vi "FitLinear2 (SubVI).vi"(0 "x values":dbl[](array[numeric]), 1 "y values":dbl[](array[numeric]), 2 "delta y values":dbl[](array[numeric]), 4 "confidence level":dbl=0.95, 5 "error in":errorcluster, 6 "Use all points":bool, 7 "Estimated centre":dbl, 8 "Fit method":T1 items=["Least Square", "Least Absolute Residual", "Bisquare"], 9 "Estimated width":dbl, 10 "Fit parameter bounds":T2={"slope min"=-inf, "slope max"=inf, "intercept min"=-inf, "intercept max"=inf}, 11 "Nsigma Low":dbl=4.0 format="%#_13g", 13 "Nsigma High":dbl=4.0 format="%#_13g") -> (14 "slope":dbl, 15 "delta slope":dbl, 16 "intercept":dbl, 17 "delta intercept":dbl, 18 "Plot with linear fit":T3(graph), 19 "error out":errorcluster)   [LabVIEW 2016]
uses:
  <vilib>/Analysis/6fits.llb/Curve Fitting Criteria.ctl
  <vilib>/Analysis/6fits.llb/Confidence Interval (Linear).vi
  <vilib>/Analysis/NI_AALPro.lvlib
panel:
  out "Best Linear Fit":dbl[](array[numeric])
  out "Selected y values":dbl[](array[numeric])
  out "Selected x values":dbl[](array[numeric])
  out "Selected delta y values":dbl[](array[numeric])
  out "residue":dbl
  # "RESULTS"
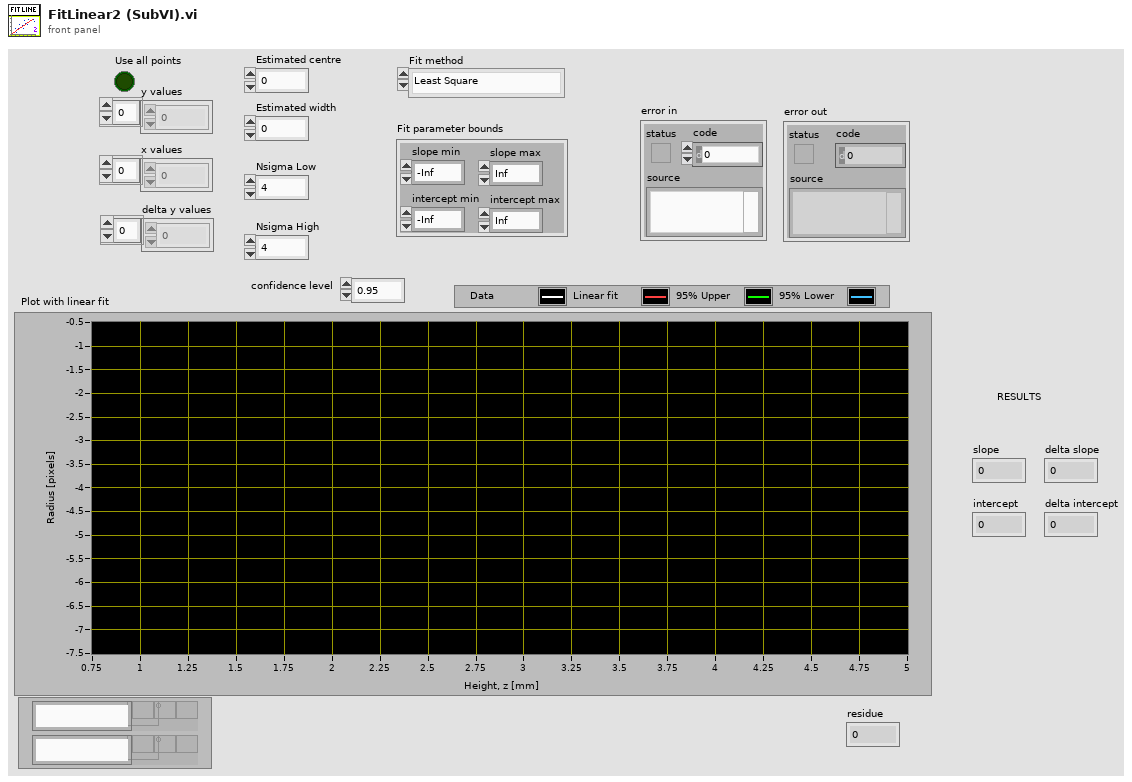
[diagram p1: front panel]
types:
  T1 = typedef "NI_AALPro.lvlib/Curve Fitting Criteria.ctl" = u16
  T2 = cluster{"slope min":dbl, "slope max":dbl, "intercept min":dbl, "intercept max":dbl}
  T3 = cluster{"Radius bins":dbl[], "Best Gaussian Fit":dbl[]}[]
  T4 = cluster{"Selected x values":dbl[], "Selected y values":dbl[]}
  T5 = cluster{"Selected x values":dbl[], "Best Linear Fit":dbl[]}
  T6 = cluster{"Selected x values":dbl[], "Upper Bound":dbl[]}
  T7 = cluster{"Selected x values":dbl[], "Lower Bound":dbl[]}
  T8 = cluster{"Selected x values":dbl[], "Lower Bound":dbl[]}[]
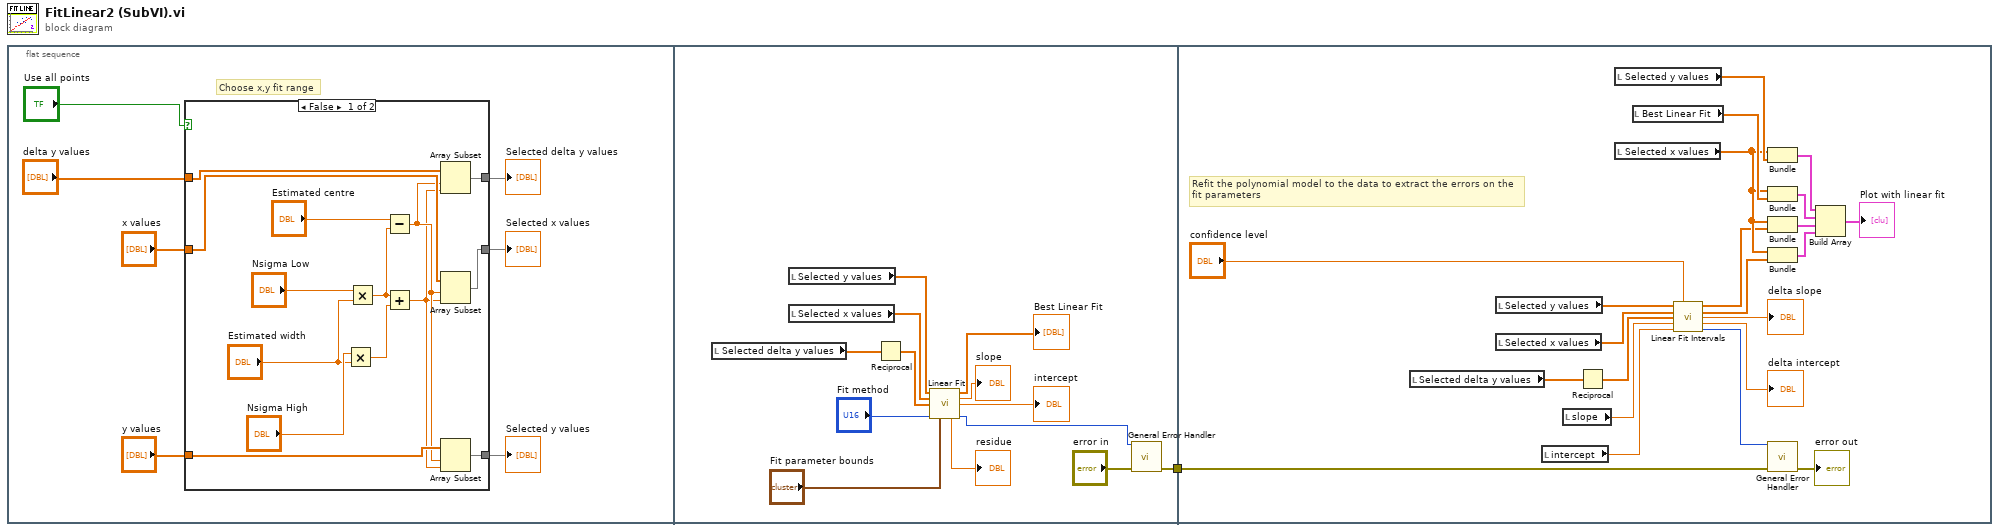
[diagram p0: block diagram]
diagram:
  n1 = flat-sequence {
    tunnel: [w38] -> w1
    tunnel: w1 -> [w51]
    frame #0 {
      # "Choose x,y fit range"
      n2 = case shown="False" "Use all points" {
        tunnel: "y values" -> [w20 w24]
        tunnel: [w19 w24] -> w4
        tunnel: "x values" -> [w18 w25]
        tunnel: [w17 w25] -> w5
        tunnel: "delta y values" -> [w12 w23]
        tunnel: [w9 w23] -> w2
        frame False {
          n3 = Multiply(x="Nsigma High", y="Estimated width") -> (x*y=w13:dbl)
          n4 = Multiply(x="Nsigma Low", y="Estimated width") -> (x*y=w14:dbl)
          n5 = Subtract(x="Estimated centre", y=w14) -> (x-y=w11:dbl)
          n6 = Add(x=w14, y=w13) -> (x+y=w10:dbl)
          n7 = Array Subset(array=w12, index=w11, length=w10) -> (w9:dbl[])
          n8 = Array Subset(array=w18, index=w11, length=w10) -> (w17:dbl[])
          n9 = Array Subset(array=w20, index=w11, length=w10) -> (w19:dbl[])
        }
        frame True {
        }
      }
      "Selected y values" <- w4
      "Selected x values" <- w5
      "Selected delta y values" <- w2
    }
    frame #1 {
      n10 = local read "Selected delta y values"() -> (w27:dbl[])
      n11 = local read "Selected y values"() -> (w29:dbl[])
      n12 = local read "Selected x values"() -> (w28:dbl[])
      n13 = Reciprocal(x=w27) -> (1/x=w26:dbl[])
      n14 = call <vilib>:"Linear Fit.vi"("Y"=w29, "X"=w28, "Weight"=w26, "method"="Fit method", "parameter bounds"="Fit parameter bounds") -> ("Best Linear Fit"=→"Best Linear Fit":dbl[], "slope"=→"slope":dbl, "intercept"=→"intercept":dbl, "residue"=→"residue":dbl, "error"=w32:i32)  [unwired: 6 in]
      n15 = call <vilib>:"General Error Handler.vi"("[error code] (0)"=w32, "error in (no error)"="error in") -> ("error out"=w38:errorcluster)  [unwired: 9 in, 4 out]
    }
    frame #2 {
      # "Refit the polynomial model to the data to extract the errors on the\nfit parameters"
      n16 = local read "Selected delta y values"() -> (w39:dbl[])
      n17 = local read "Selected y values"() -> (w50:dbl[])
      n18 = local read "Selected x values"() -> (w49:dbl[])
      n19 = local read "intercept"() -> (w47:dbl)
      n20 = local read "slope"() -> (w48:dbl)
      n21 = Reciprocal(x=w39) -> (1/x=w40:dbl[])
      n22 = local read "Selected y values"() -> (w59:dbl[])
      n23 = local read "Selected x values"() -> (w56:dbl[])
      n24 = local read "Best Linear Fit"() -> (w58:dbl[])
      n25 = call-poly <vilib>:"Linear Fit Intervals.vi"("Y"=w50, "confidence level"="confidence level", "X"=w49, "Weight"=w40, "slope"=w48, "intercept"=w47) -> ("Upper Bound"=w44:dbl[], "Lower Bound"=w45:dbl[], "delta slope"=→"delta slope":dbl, "delta intercept"=→"delta intercept":dbl, "error"=w46:i32)  [unwired: 5 in]
      n26 = Bundle("Selected x values"=w56, "Selected y values"=w59) -> (w57:T4)  [unwired: 1 in]
      n27 = Bundle("Selected x values"=w56, "Best Linear Fit"=w58) -> (w55:T5)  [unwired: 1 in]
      n28 = Bundle("Selected x values"=w56, "Upper Bound"=w44) -> (w54:T6)  [unwired: 1 in]
      n29 = Bundle("Selected x values"=w56, "Lower Bound"=w45) -> (w53:T7)  [unwired: 1 in]
      n30 = call <vilib>:"General Error Handler.vi"("[error code] (0)"=w46, "error in (no error)"=w51) -> ("error out"=→"error out":errorcluster)  [unwired: 9 in, 4 out]
      n31 = Build Array(w57, w55, w54, w53) -> (→"Plot with linear fit":T8)
    }
  }
